vi "Set Intensity Graph Scales (Start and End).vi"(8 "error in (no error)":errorcluster, 9 "y start & end":cluster{"y start":dbl, "y end":dbl}, 10 "x start & end":cluster{"x start":dbl, "x end":dbl}, 11 "graph_utilities in":refnum<class "graph_utilities.lvclass">) -> (0 "error out":errorcluster, 3 "graph_utilities out":refnum<class "graph_utilities.lvclass">)   [LabVIEW 2020, in "graph_utilities.lvclass"]
uses:
  graph_utilities.lvclass
  <vilib>/Utility/miscctls.llb/LVOffsetAndMultiplierTypeDef.ctl
  graph_utilities.lvclass/graph_utilities.ctl
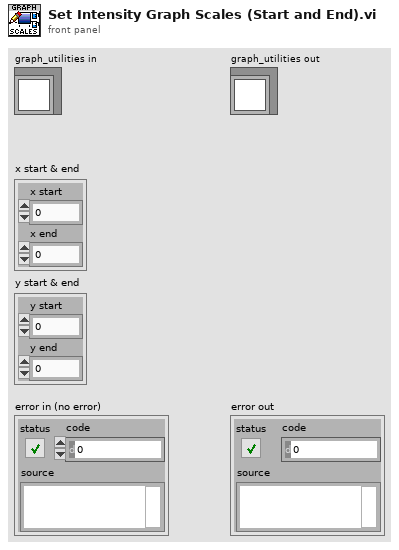
[diagram p1: front panel]
types:
  T1 = typedef "LVOffsetAndMultiplierTypeDef.ctl" = cluster{"Offset":dbl, "Multiplier":dbl}
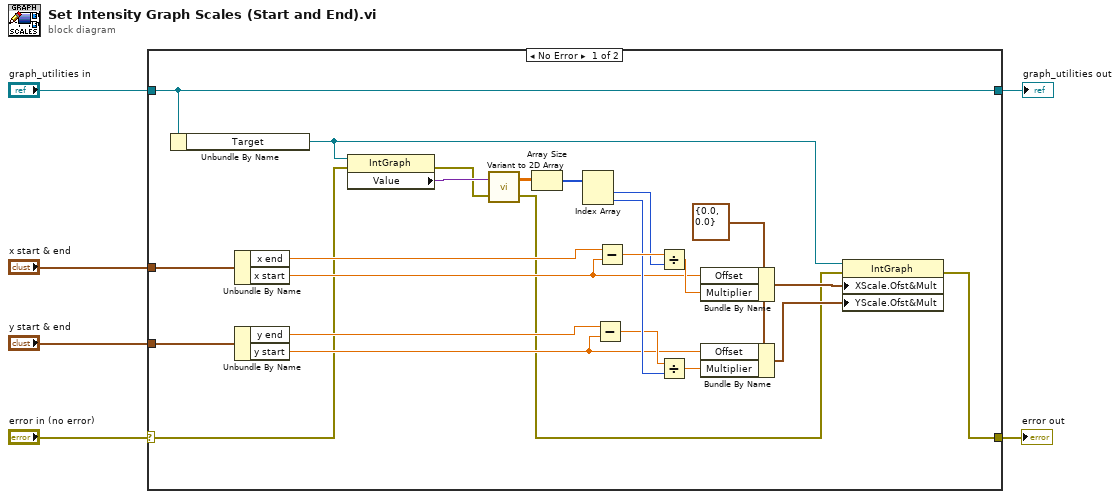
[diagram p0: block diagram]
diagram:
  n1 = case shown="No Error" "error in (no error)" {
    selector: "error in (no error)" -> [w9 w32]
    tunnel: "x start & end" -> [w27 _]
    tunnel: "y start & end" -> [w25 _]
    tunnel: [w20 w32] -> w4
    tunnel: "graph_utilities in" -> [w14 w31]
    tunnel: [w14 w31] -> w1
    frame No Error {
      w21 = T1 {"Offset"=0.0, "Multiplier"=0.0} ("X Scale.Offset and Multiplier")
      n2 = Unbundle By Name(w14) -> ("Target"=w11:refnum<vi>)
      n3 = Unbundle By Name(w27) -> ("x end"=w26:dbl, "x start"=w17:dbl)
      n4 = Unbundle By Name(w25) -> ("y end"=w24:dbl, "y start"=w15:dbl)
      n5 = property on="Property Node" class="IntGraph"(reference=w11, error in=w9) -> (error out=w12:errorcluster, "Value"=w13:variant)  [unwired: 1 out]
      n6 = call "Variant to 2D Array.vi"("error in (no error)"=w12, "Value"=w13) -> ("error out"=w8:errorcluster, "Array"=w10:dbl[][])
      n7 = Array Size(array=w10) -> (size(s)=w7:i32[])
      n8 = Index Array(array=w7) -> (element #1=w18:i32, element #2=w23:i32)  [unwired: 2 in]
      n9 = Subtract(x=w24, y=w15) -> (x-y=w16:dbl)
      n10 = Subtract(x=w26, y=w17) -> (x-y=w28:dbl)
      n11 = Divide(x=w28, y=w18) -> (x/y=w19:dbl)
      n12 = Divide(x=w16, y=w23) -> (x/y=w29:dbl)
      n13 = Bundle By Name(cluster=w21, "Offset"=w17, "Multiplier"=w19) -> (w30:T1)
      n14 = Bundle By Name(cluster=w21, "Offset"=w15, "Multiplier"=w29) -> (w22:T1)
      n15 = property on="Property Node" class="IntGraph"(reference=w11, error in=w8, "XScale.Ofst&Mult"=w30, "YScale.Ofst&Mult"=w22) -> (error out=w20:errorcluster)  [unwired: 1 out]
    }
    frame Error {
    }
  }
  "error out" <- w4
  "graph_utilities out" <- w1
